vi "Query Instruments.vi"(8 "error in":errorcluster, 10 "Instrument Notifier":refnum<notifier>, 11 "Base Software in":refnum<class "Main.lvclass">) -> (0 "error out":errorcluster, 3 "Base Software out":refnum<class "Main.lvclass">)   [LabVIEW 2023, in "Main.lvlib" / "Main.lvclass"]
uses:
  Project/Main.lvclass
  builds/Engine/Actor Framework.lvlibp/1abvi3w/vi.lib/ActorFramework/Message Enqueuer/Message Enqueuer.lvclass
  Custom Controls/g_Identifiers.vi
  builds/Base Software/Panels/Manual UI.lvlibp/Manual UI Messages/Query Instruments Msg/Query Instruments Msg.lvclass
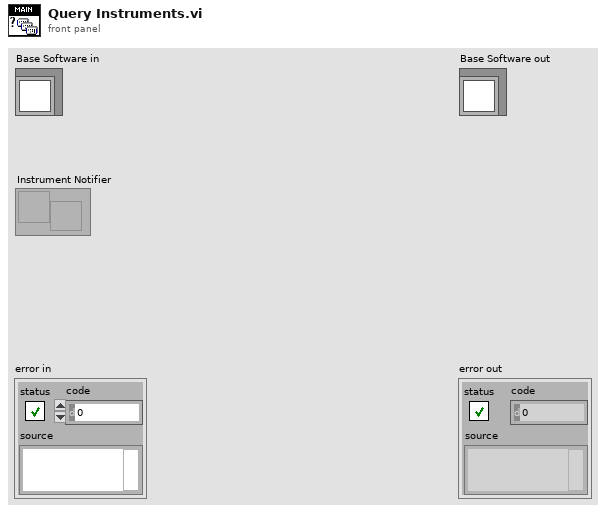
[diagram p1: front panel]
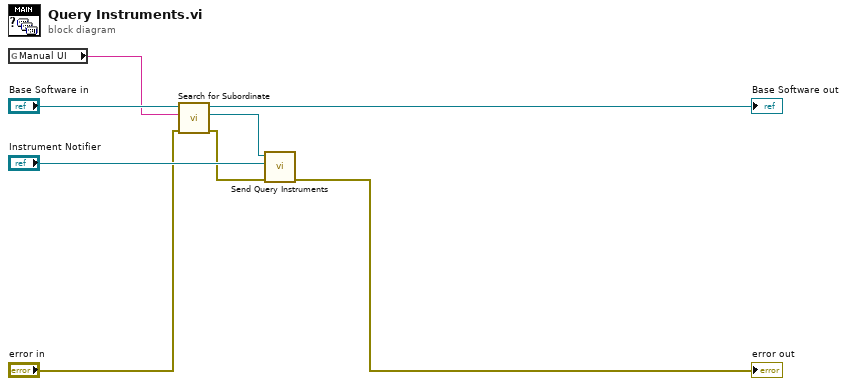
[diagram p0: block diagram]
diagram:
  n1 = global read "g_Identifiers.vi" "Manual UI"() -> (w7:string)
  n2 = call "Search for Subordinate.vi"("error in"="error in", "Identifier"=w7, "Base Software in"="Base Software in") -> ("error out"=w3:errorcluster, "Enqueuer"=w6:refnum<class "Message Enqueuer.lvclass">, "Base Software out"=→"Base Software out":refnum<class "Main.lvclass">)  [unwired: 3 in, 3 out]
  n3 = call "Send Query Instruments.vi"("error in (no error)"=w3, "Instrument Notifier"="Instrument Notifier", "Message Enqueuer"=w6) -> ("error out"=→"error out":errorcluster)  [unwired: 7 in, 1 out]
